vi "ParseSerial2JSON.vi"(6 "Function":enum16{"Serial", "Unserial"}(ring)=enum."Unserial", 8 "error in (no error)":errorcluster, 10 "Array":T1(array[cluster]), 11 "input":string) -> (0 "error out":errorcluster, 2 "string out":string, 3 "output":T2)   [LabVIEW 2014]
panel:
  out "result string":string
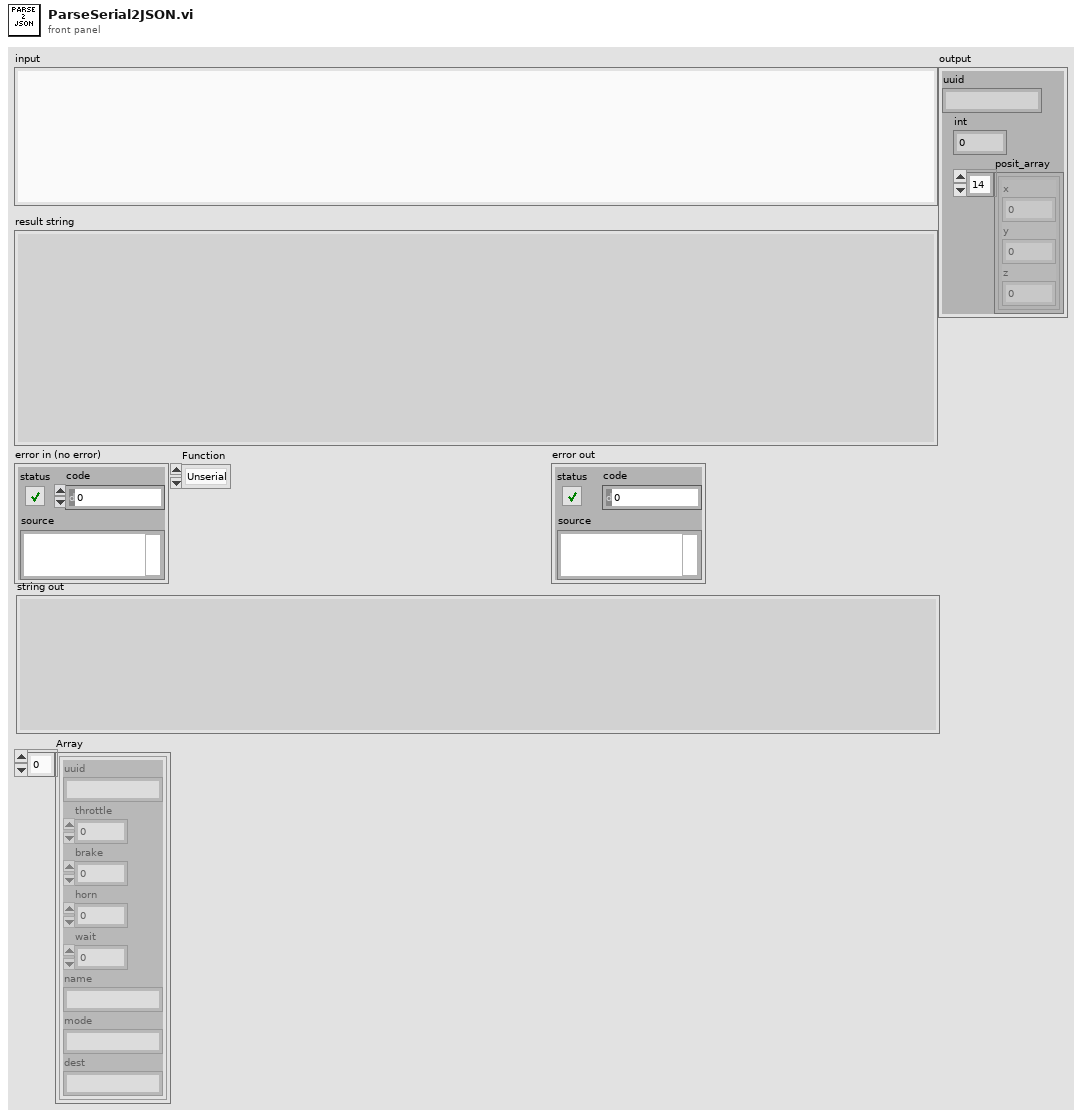
[diagram p1: front panel]
types:
  T1 = cluster{"uuid":string, "throttle":dbl, "brake":dbl, "horn":dbl, "wait":dbl, "name":string, "mode":string, "dest":string}[]
  T2 = cluster{"uuid":string, "int":i32, "posit_array":cluster{"x":dbl, "y":dbl, "z":dbl}[]}
  T3 = cluster{"0":string, "1":dbl, "2":dbl, "3":dbl, "4":dbl, "5":string, "6":string, "7":string}
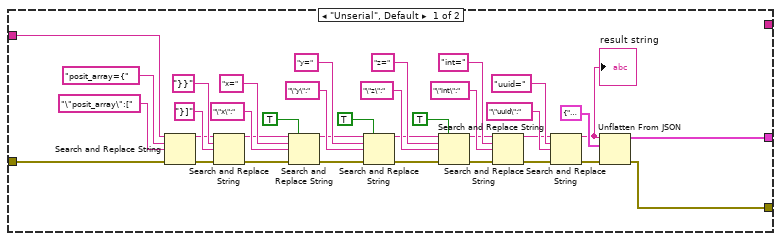
[diagram p2: hidden frame]
diagram:
  (unwired) T3 {"0"="", "1"=0.0, "2"=0.0, "3"=0.0, "4"=0.0, "5"="", "6"="", "7"=""} ("train_control")
  # "{{[\"1\"]=0.34221,[\"0\"]=\"28badb08-2150-49dc-b2b3-446ab3bd8db5\",[\"3\"]=0,[\"2\"]=0.65779,[\"5\"]=\"T25\",[\"4\"]=0.5,[\"7\"]=\"Station2\",[\"6\"]=\"Station Timer\"},{[\"1\"]=0,[\"0\"]=\"0d9dd51e-9eb0-4643-b1ca-17aa2bbef216\",[\"3\"]=0,[\"2\"]=1,[\"5\"]=\"T17\",[\"4\"]=0.5,[\"7\"]=\"Station2\",[\"6\"]=\"Station Timer\"},{[\"1\"]=0,[\"0\"]=\"7500b925-bb53-45af-a409-00a653106864\",[\"3\"]=0,[\"2\"]=1,[\"5\"]=\"T21\",[\"4\"]=0.5,[\"7\"]=\"Station2\",[\"6\"]=\"Station Timer\"},{[\"1\"]=0.1188,[\"0\"]=\"4cfdd4c6-2eba-4f44-a429-3244b5bb652a\",[\"3\"]=0,[\"2\"]=0.8812,[\"5\"]=\"T20\",[\"4\"]=0.5,[\"7\"]=\"Station2\",[\"6\"]=\"Station Timer\"},{[\"1\"]=0,[\"0\"]=\"8d575721-4606-4466-b498-e7b32d22f971\",[\"3\"]=0,[\"2\"]=1,[\"5\"]=\"T27\",[\"4\"]=0.5,[\"7\"]=\"Station2\",[\"6\"]=\"Station Timer\"},{[\"1\"]=0.242,[\"0\"]=\"8186529a-1635-439f-8295-aa55fffa2b03\",[\"3\"]=0,[\"2\"]=0.758,[\"5\"]=\"T28\",[\"4\"]=0.5,[\"7\"]=\"Station2\",[\"6\"]=\"Station Timer\"},{[\"1\"]=0.242,[\"0\"]=\"7bf20173-7541-4e2c-b414-3a497e915463\",[\"3\"]=0,[\"2\"]=0.758,[\"5\"]=\"T19\",[\"4\"]=0.5,[\"7\"]=\"Station2\",[\"6\"]=\"Station Timer\"},{[\"1\"]=0.242,[\"0\"]=\"d798c515-e8fd-414b-a7d0-03bacc84b7f2\",[\"3\"]=0,[\"2\"]=0.758,[\"5\"]=\"T32\",[\"4\"]=0.5,[\"7\"]=\"Station2\",[\"6\"]=\"Station Timer\"},{[\"1\"]=0.0374,[\"0\"]=\"f96f55ad-fa64-4c46-83e7-01e7ceff0553\",[\"3\"]=0,[\"2\"]=0.9626,[\"5\"]=\"T29\",[\"4\"]=0.5,[\"7\"]=\"Station2\",[\"6\"]=\"Station Timer\"},{[\"1\"]=-2,[\"0\"]=\"fe1e82df-d2b2-4655-ab6f-589ae6b23eba\",[\"3\"]=-2,[\"2\"]=-2,[\"5\"]=\"T1\",[\"4\"]=0.5,[\"7\"]=\"\",[\"6\"]=\"Tracker\"},{[\"1\"]=0.2618,[\"0\"]=\"4347b93f-ea48-4aca-ad50-6ef407a024e0\",[\"3\"]=0,[\"2\"]=0.7382,[\"5\"]=\"T30\",[\"4\"]=0.5,[\"7\"]=\"Station2\",[\"6\"]=\"Station Timer\"},{[\"1\"]=0.1496,[\"0\"]=\"397c125a-0f82-495d-bdde-342d563b00bd\",[\"3\"]=0,[\"2\"]=0.8504,[\"5\"]=\"T24\",[\"4\"]=0.5,[\"7\"]=\"Station2\",[\"6\"]=\"Station Timer\"},{[\"1\"]=0,[\"0\"]=\"6c309be4-fa62-4890-906a-955d3ac1c4a0\",[\"3\"]=0,[\"2\"]=1,[\"5\"]=\"T23\",[\"4\"]=0.5,[\"7\"]=\"Station2\",[\"6\"]=\"Station Timer\"},{[\"1\"]=0.26587,[\"0\"]=\"4e535d14-e610-4486-8a4b-cef48708d7a8\",[\"3\"]=0,[\"2\"]=0.73413,[\"5\"]=\"T26\",[\"4\"]=0.5,[\"7\"]=\"Station2\",[\"6\"]=\"Station Timer\"},{[\"1\"]=0,[\"0\"]=\"fe410c57-7fcd-462f-835d-7cdf641e4f6e\",[\"3\"]=0,[\"2\"]=1,[\"5\"]=\"T22\",[\"4\"]=0.5,[\"7\"]=\"Station2\",[\"6\"]=\"Station Timer\"},{[\"1\"]=0,[\"0\"]=\"6e880836-fff2-40c1-994d-e1218dc8e61c\",[\"3\"]=0,[\"2\"]=1,[\"5\"]=\"T18\",[\"4\"]=0.5,[\"7\"]=\"Station2\",[\"6\"]=\"Station Timer\"}}"
  # "[{\"uuid\":\"0d9dd51e-9eb0-4643-b1ca-17aa2bbef216\",\"throttle\":0,\"brake\":1,\"horn\":0,\"wait\":0.5,\"name\":\"T17\",\"mode\":\"Maintain\",\"dest\":\"\"},{\"uuid\":\"ace6ad33-5ccf-4a11-8aae-eab4bf9e4ae7\",\"throttle\":-2,\"brake\":-2,\"horn\":-2,\"wait\":5,\"name\":\"T12\",\"mode\":\"Manual\",\"dest\":\"\"},{\"uuid\":\"2294d077-d4be-4cc2-8fce-0b4721cfc771\",\"throttle\":-2,\"brake\":-2,\"horn\":-2,\"wait\":5,\"name\":\"T15\",\"mode\":\"Manual\",\"dest\":\"\"},{\"uuid\":\"716a234a-9df1-40a7-a466-2ea33ed7dd6a\",\"throttle\":-2,\"brake\":-2,\"horn\":-2,\"wait\":5,\"name\":\"T6\",\"mode\":\"Manual\",\"dest\":\"\"},{\"uuid\":\"27faf7eb-c562-4e80-a598-b4ac4d39b456\",\"throttle\":-2,\"brake\":-2,\"horn\":-2,\"wait\":5,\"name\":\"T10\",\"mode\":\"Manual\",\"dest\":\"\"},{\"uuid\":\"fe1e82df-d2b2-4655-ab6f-589ae6b23eba\",\"throttle\":0,\"brake\":1,\"horn\":0,\"wait\":0.5,\"name\":\"T31\",\"mode\":\"Maintain\",\"dest\":\"\"},{\"uuid\":\"333f5dec-454f-48ed-9f99-6d55c8118ae9\",\"throttle\":-2,\"brake\":-2,\"horn\":-2,\"wait\":5,\"name\":\"T5\",\"mode\":\"Manual\",\"dest\":\"\"},{\"uuid\":\"4e535d14-e610-4486-8a4b-cef48708d7a8\",\"throttle\":0,\"brake\":1,\"horn\":0,\"wait\":0.5,\"name\":\"T26\",\"mode\":\"Maintain\",\"dest\":\"\"},{\"uuid\":\"4347b93f-ea48-4aca-ad50-6ef407a024e0\",\"throttle\":0.55032347124207126,\"brake\":0.44967652875792874,\"horn\":0,\"wait\":0.5,\"name\":\"T30\",\"mode\":\"Maintain\",\"dest\":\"\"},{\"uuid\":\"397c125a-0f82-495d-bdde-342d563b00bd\",\"throttle\":0.11245814275610508,\"brake\":0.88754185724389489,\"horn\":0,\"wait\":0.5,\"name\":\"T24\",\"mode\":\"Maintain\",\"dest\":\"\"},{\"uuid\":\"7bf20173-7541-4e2c-b414-3a497e915463\",\"throttle\":0.16386677777777575,\"brake\":0.83613322222222419,\"horn\":0,\"wait\":0.5,\"name\":\"T19\",\"mode\":\"Maintain\",\"dest\":\"\"},{\"uuid\":\"8186529a-1635-439f-8295-aa55fffa2b03\",\"throttle\":0,\"brake\":1,\"horn\":0,\"wait\":0.5,\"name\":\"T28\",\"mode\":\"Maintain\",\"dest\":\"\"},{\"uuid\":\"86639eaf-f0ee-4829-8a22-b1670cdc2141\",\"throttle\":-2,\"brake\":-2,\"horn\":-2,\"wait\":5,\"name\":\"T14\",\"mode\":\"Manual\",\"dest\":\"\"},{\"uuid\":\"aa77cf07-dd73-4f5f-83c1-193bed907ca8\",\"throttle\":-2,\"brake\":-2,\"horn\":-2,\"wait\":5,\"name\":\"T11\",\"mode\":\"Manual\",\"dest\":\"\"},{\"uuid\":\"4cfdd4c6-2eba-4f44-a429-3244b5bb652a\",\"throttle\":0,\"brake\":1,\"horn\":0,\"wait\":0.5,\"name\":\"T20\",\"mode\":\"Maintain\",\"dest\":\"\"},{\"uuid\":\"cb33e381-b194-4042-b84a-1c3298ce8b24\",\"throttle\":-2,\"brake\":-2,\"horn\":-2,\"wait\":5,\"name\":\"T13\",\"mode\":\"Manual\",\"dest\":\"\"},{\"uuid\":\"28badb08-2150-49dc-b2b3-446ab3bd8db5\",\"throttle\":0.11239677410082553,\"brake\":0.88760322589917451,\"horn\":0,\"wait\":0.5,\"name\":\"T25\",\"mode\":\"Maintain\",\"dest\":\"\"},{\"uuid\":\"d798c515-e8fd-414b-a7d0-03bacc84b7f2\",\"throttle\":0,\"brake\":1,\"horn\":0,\"wait\":0.5,\"name\":\"T32\",\"mode\":\"Maintain\",\"dest\":\"\"},{\"uuid\":\"f96f55ad-fa64-4c46-83e7-01e7ceff0553\",\"throttle\":0.80000000000000004,\"brake\":0.014008277777778355,\"horn\":0,\"wait\":0.5,\"name\":\"T29\",\"mode\":\"Maintain\",\"dest\":\"\"},{\"uuid\":\"fe410c57-7fcd-462f-835d-7cdf641e4f6e\",\"throttle\":0,\"brake\":1,\"horn\":0,\"wait\":0.5,\"name\":\"T22\",\"mode\":\"Maintain\",\"dest\":\"\"},{\"uuid\":\"6457e477-1b75-4671-93e9-0f9b5a45e000\",\"throttle\":-2,\"brake\":-2,\"horn\":-2,\"wait\":5,\"name\":\"T4\",\"mode\":\"Manual\",\"dest\":\"\"},{\"uuid\":\"fcc7feed-1001-4c94-85e0-4a2196553b2c\",\"throttle\":0,\"brake\":1,\"horn\":0,\"wait\":0.5,\"name\":\"T16\",\"mode\":\"Maintain\",\"dest\":\"\"},{\"uuid\":\"4980fb9d-d4c0-4abf-ae21-9f8c3ad2105c\",\"throttle\":-2,\"brake\":-2,\"horn\":-2,\"wait\":0.5,\"name\":\"T1\",\"mode\":\"Tracker\",\"dest\":\"\"},{\"uuid\":\"6e880836-fff2-40c1-994d-e1218dc8e61c\",\"throttle\":0.10666072663431418,\"brake\":0.89333927336568586,\"horn\":0,\"wait\":0.5,\"name\":\"T18\",\"mode\":\"Maintain\",\"dest\":\"\"},{\"uuid\":\"6c309be4-fa62-4890-906a-955d3ac1c4a0\",\"throttle\":0,\"brake\":1,\"horn\":0,\"wait\":0.5,\"name\":\"T23\",\"mode\":\"Maintain\",\"dest\":\"\"},{\"uuid\":\"7500b925-bb53-45af-a409-00a653106864\",\"throttle\":0.0060652777777782932,\"brake\":0.99393472222222168,\"horn\":0,\"wait\":0.5,\"name\":\"T21\",\"mode\":\"Maintain\",\"dest\":\"\"},{\"uuid\":\"345f635b-f040-4fad-afe2-09000f9fc1ea\",\"throttle\":-2,\"brake\":-2,\"horn\":-2,\"wait\":5,\"name\":\"T3\",\"mode\":\"Manual\",\"dest\":\"\"},{\"uuid\":\"a88afee6-40e5-4e97-8a54-a7531d5122dd\",\"throttle\":-2,\"brake\":-2,\"horn\":-2,\"wait\":5,\"name\":\"T7\",\"mode\":\"Manual\",\"dest\":\"\"},{\"uuid\":\"8d575721-4606-4466-b498-e7b32d22f971\",\"throttle\":0.80000000000000004,\"brake\":0.022014166666665891,\"horn\":0,\"wait\":0.5,\"name\":\"T27\",\"mode\":\"Maintain\",\"dest\":\"\"}]"
  # "{\"uuid\":\"abc\",\"int\":1,\"posit_array\":[{\"x\":1,\"y\":2,\"z\":3},{\"x\":4,\"y\":5,\"z\":6}]}"
  # "{posit_array={{z=-353.5,x=1161.912,y=64.051},{z=-353.5,x=1161.912,y=64.051},{z=-353.5,x=1161.912,y=64.051},\n{z=-353.5,x=1161.912,y=64.051},{z=-353.5,x=1161.912,y=64.051},{z=-353.5,x=1161.912,y=64.051},{z=-353.5,x=1161.912,y=64.051},\n{z=-353.5,x=1161.912,y=64.051},{z=-353.5,x=1161.912,y=64.051},{z=-353.5,x=1161.912,y=64.051},{z=-353.5,x=1161.912,y=64.051},\n{z=-353.5,x=1161.912,y=64.051},{z=-353.5,x=1161.912,y=64.051},{z=-353.5,x=1161.912,y=64.051},{z=-353.5,x=1161.912,y=64.051}},\nuuid=\"4cfdd4c6-2eba-4f44-a429-3244b5bb652a\",nt=1}"
  n1 = case shown="\"Serial\"" "Function" {
    tunnel: "input" -> [w20 _]
    tunnel: [w17 _] -> w6
    tunnel: [w9 w58] -> w5
    tunnel: "error in (no error)" -> [w8 w59]
    tunnel: [_ w57] -> w2
    tunnel: "Array" -> [_ w44]
    frame "Unserial", Default {
      n2 = Search and Replace String(input string=w20, search string="posit_array={", replace string="\"posit_array\":[" ("replace string (\"\")"), error in=w8) -> (result string=w26:string, error out=w10:errorcluster)  [unwired: 4 in, 2 out]
      n3 = Search and Replace String(input string=w26, search string="}}", replace string="}]" ("replace string (\"\")"), error in=w10) -> (result string=w25:string, error out=w11:errorcluster)  [unwired: 4 in, 2 out]
      n4 = Search and Replace String(replace all?=TRUE ("replace all? (F)"), input string=w25, search string="x=", replace string="\"x\":" ("replace string (\"\")"), error in=w11) -> (result string=w24:string, error out=w12:errorcluster)  [unwired: 3 in, 2 out]
      n5 = Search and Replace String(replace all?=TRUE ("replace all? (F)"), input string=w24, search string="y=", replace string="\"y\":" ("replace string (\"\")"), error in=w12) -> (result string=w23:string, error out=w13:errorcluster)  [unwired: 3 in, 2 out]
      n6 = Search and Replace String(replace all?=TRUE ("replace all? (F)"), input string=w23, search string="z=", replace string="\"z\":" ("replace string (\"\")"), error in=w13) -> (result string=w22:string, error out=w14:errorcluster)  [unwired: 3 in, 2 out]
      n7 = Search and Replace String(input string=w22, search string="int=", replace string="\"int\":" ("replace string (\"\")"), error in=w14) -> (result string=w21:string, error out=w15:errorcluster)  [unwired: 4 in, 2 out]
      n8 = Search and Replace String(input string=w21, search string="uuid=", replace string="\"uuid\":" ("replace string (\"\")"), error in=w15) -> (result string=w18:string, error out=w16:errorcluster)  [unwired: 4 in, 2 out]
      "result string" <- w18
      n9 = Unflatten From JSON(JSON string=w18, type and defaults=T2 {"uuid"="", "int"=0, "posit_array"=[]} ("train_data"), error in (no error)=w16) -> (value=w17:T2, error out=w9:errorcluster)  [unwired: 4 in]
    }
    frame "Serial" {
      n10 = for {
        tunnel: w44 -> [w71] mode=indexing
        tunnel: [w62] -> w45 mode=indexing
        n11 = Unbundle(w71) -> ("uuid"=w63:string, "throttle"=w64:dbl, "brake"=w65:dbl, "horn"=w66:dbl, "wait"=w67:dbl, "name"=w68:string, "mode"=w69:string, "dest"=w70:string)
        n12 = Bundle(cluster=T3 {"0"="", "1"=0.0, "2"=0.0, "3"=0.0, "4"=0.0, "5"="", "6"="", "7"=""} ("train_control"), "0"=w63, "1"=w64, "2"=w65, "3"=w66, "4"=w67, "5"=w68, "6"=w69, "7"=w70) -> (w62:T3)
      }
      n13 = Flatten To JSON(enable LabVIEW extensions? (T)=FALSE, anything=w45, error in (no error)=w59) -> (JSON string=w52:string, 11:w46:errorcluster)
      n14 = Search and Replace String(input string=w52, search string="[{" ("replace string (\"\")"), replace string="{{" ("search string"), error in=w46) -> (result string=w50:string, error out=w49:errorcluster)  [unwired: 4 in, 2 out]
      n15 = for {
        tunnel: string[] ["0", "1", "2", "3", "4", "5", "6", "7"] -> [w78] mode=indexing
        shift-right: [w80] -> w48
        shift-left: w50 -> [w81]
        shift-right: [w73] -> w47
        shift-left: w49 -> [w74]
        w83 = "\"" ("string")
        n16 = Concatenate Strings(w83, w78, w83, ":" ("string")) -> (w75:string)
        n17 = Concatenate Strings("[\"" ("string"), w78, "\"]=" ("string")) -> (w76:string)
        n18 = Search and Replace String(replace all?=TRUE ("replace all? (F)"), input string=w81, search string=w75, replace string=w76, error in=w74) -> (result string=w80:string, error out=w73:errorcluster)  [unwired: 3 in, 2 out]
      }
      n19 = Search and Replace String(input string=w48, search string="}]" ("replace string (\"\")"), replace string="}}" ("search string"), error in=w47) -> (result string=w57:string, error out=w58:errorcluster)  [unwired: 4 in, 2 out]
    }
  }
  "output" <- w6
  "error out" <- w5
  "string out" <- w2
